vi "GEA2 Message to HEUI_LEDs_Idle.vi"(7 "Raw Data In":string) -> (8 "HEUI_LEDs":T1)   [LabVIEW 2016, in "TLMB.lvlib"]
uses:
  Projects/TLMB.lvlib
  controls/HEUI_LEDs.ctl
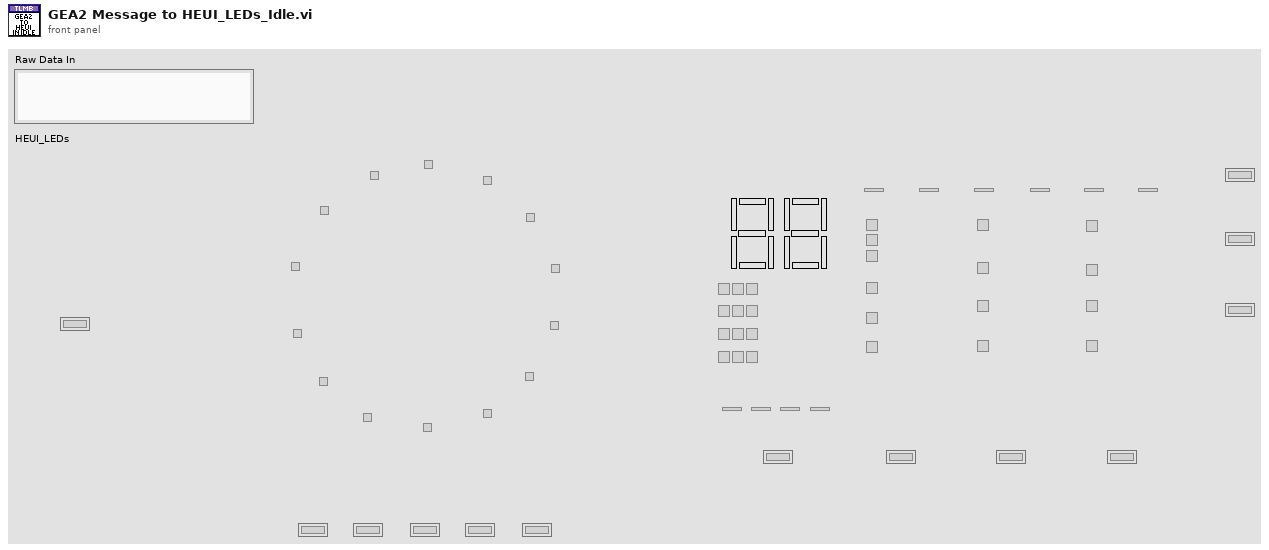
[diagram p1: front panel]
types:
  T1 = typedef "TLMB.lvlib/HEUI_LEDs.ctl" = cluster{"Z101 - Start":bool, "Z103 - Colors":bool, "Z104 - Whites":bool, "Z105 - Towels":bool, "Z106 - Bulky Items":bool, "Z107 - Heavy Duty":bool, "Z108 - Jeans":bool, "Z109 - Basket Clean":bool, "Z110 - Drain and Spin":bool, "Z111 - Rinse and Spin":bool, "Z112 - Speed Wash":bool, "Z113 - Active Wear":bool, "Z114 - Hand Wash":bool, "Z115 - Delicates":bool, "Z116 - Easy Care":bool, "Z117 - Tomato":bool, "Z118 - Wine":bool, "Z119 - Blood":bool, "Z120 - Grass":bool, "Z121 - Dirt":bool, "Z122_MSB_A":bool, "Z123_MSB_B":bool, "Z124_MSB_G":bool, "Z125_MSB_C":bool, "Z126_MSB_D":bool, "Z127_MSB_E":bool, "Z128_MSB_F":bool, "Z129_LSB_A":bool, "Z130_LSB_B":bool, "Z131_LSB_G":bool, "Z132_LSB_C":bool, "Z133_LSB_D":bool, "Z134_LSB_E":bool, "Z135_LSB_F":bool, "Z136 - Pause":bool, "Z137 - Pause":bool, "Z138 - Lock Controls":bool, "Z139 - Lock Controls":bool, "Z140 - Lock Controls":bool, "Z141 - Lid Lock":bool, "Z142 - Lid Lock":bool, "Z143 - Lid Lock":bool, "Z144 - Good":bool, "Z145":bool, "Z146":bool, "Z147 - Better":bool, "Z148 - Delay":bool, "Z149 - Fill":bool, "Z150 - Soak":bool, "Z151 - Wash":bool, "Z152 - Rinse":bool, "Z153 - Spin":bool, "Z154 - Hot":bool, "Z155 - Warm":bool, "Z156 - Colors":bool, "Z157 - Cool":bool, "Z158 - Cold":bool, "Z159 - Tap Cold":bool, "Z160 - Extra Heavy":bool, "Z161 - Heavy":bool, "Z162 - Normal":bool, "Z163 - Light":bool, "Z164 - Max Spin":bool, "Z165 - More Spin":bool, "Z166 - Normal Spin":bool, "Z167 - No Spin":bool, "Z168 - Extra Rinse":bool, "Z170 - Deep Rinse":bool, "Z171 - Auto Soak":bool, "Z172 - Warm Rinse":bool, "Z173 - Deep Fill":bool, "Z174 - My Cycles":bool, "Z175 - Delay Wash":bool, "Z176 - Spin Stop":bool, "Z177 - Spin Stop":bool, "Z178 - Spin Stop":bool, "Z179 - Pause":bool, "Z109":bool, "Z110":bool, "Z123":bool, "Z124":bool, "Z140":bool, "Unused0":bool, "Unused1":bool, "Unused2":bool, "Unused3":bool, "Channel_Off":bool, "Channel_Cycle_Unmapped":bool}
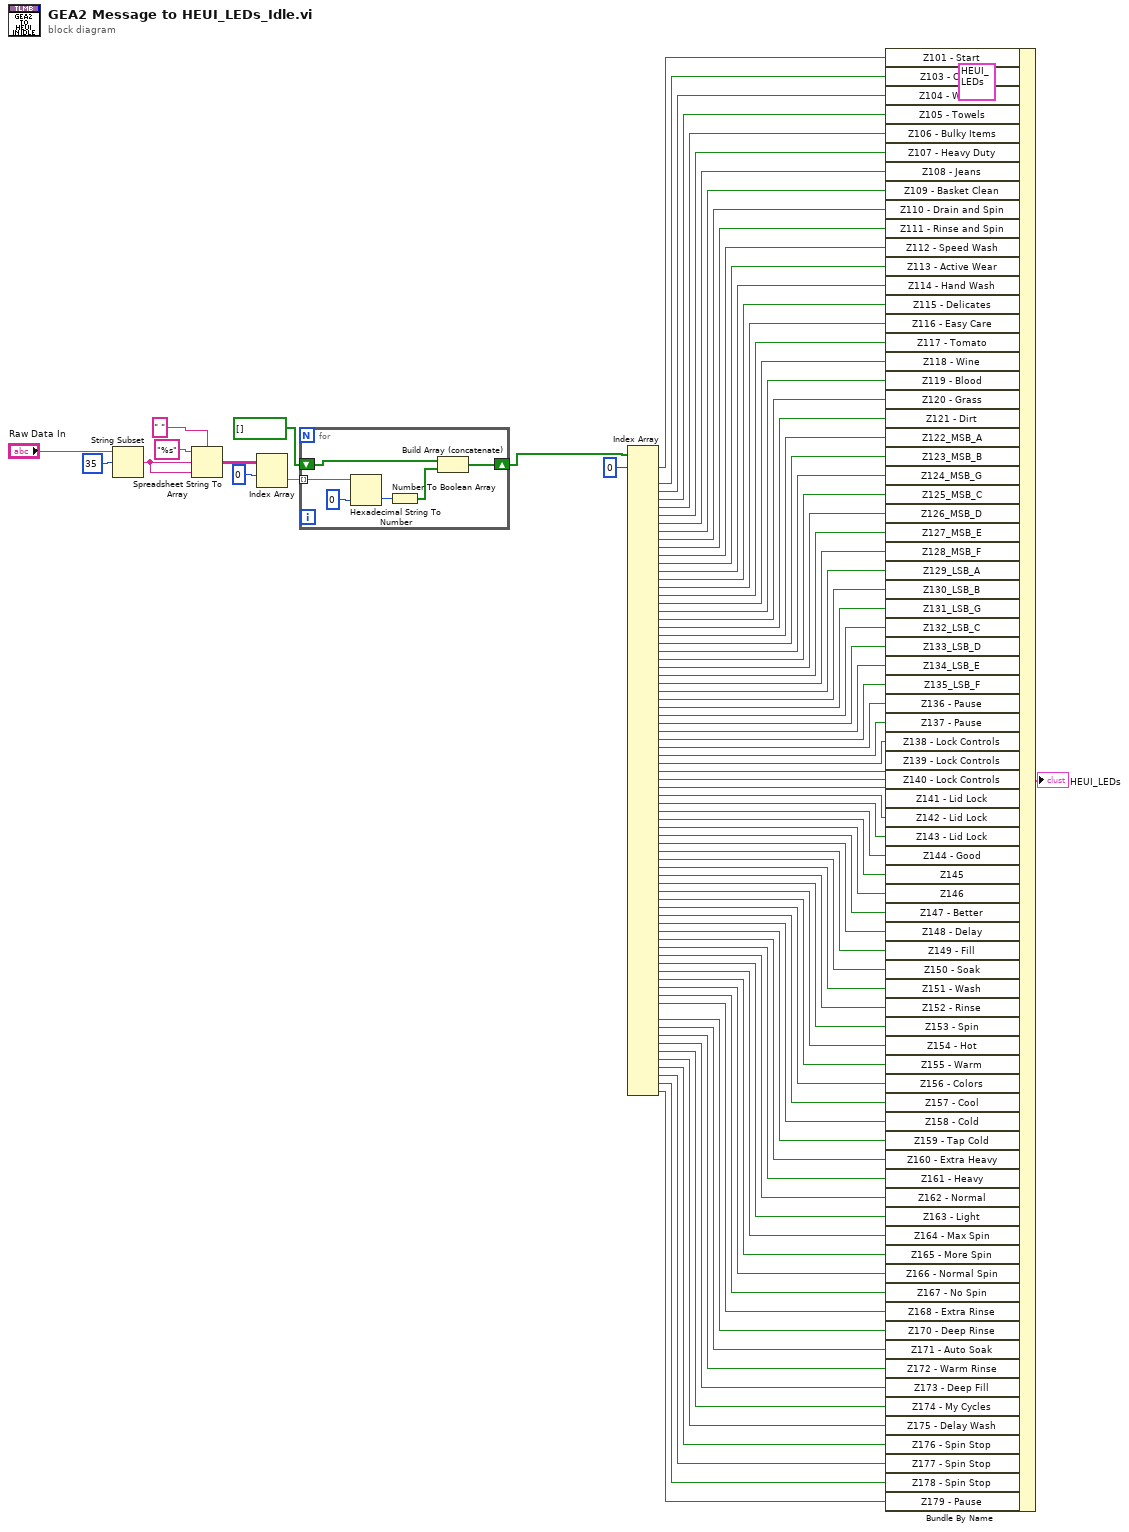
[diagram p0: block diagram]
diagram:
  n1 = String Subset(string="Raw Data In", offset (0)=35) -> (substring=w83:string)  [unwired: 1 in]
  n2 = Spreadsheet String To Array(delimiter (Tab)=" ", format string="%s", spreadsheet string=w83, array type (2D Dbl)=w83) -> (array=w87:string[][])
  n3 = Index Array(array=w87, index (row)=0) -> (element=w84:string[])  [unwired: 1 in]
  n4 = for {
    tunnel: w84 -> [w96] mode=indexing
    shift-right: [w92] -> w1
    shift-left: bool[] [] -> [w94]
    n5 = Hexadecimal String To Number(string=w96, default (0uL)=u8 0) -> (number=w95:u8)  [unwired: 1 in, 1 out]
    n6 = Number To Boolean Array(number=w95) -> (Boolean array=w93:bool[])
    n7 = Build Array (concatenate)(w94, w93) -> (w92:bool[])
  }
  n8 = Index Array(array=w1, index #1=0 ("index")) -> (element #1=w82:bool, element #3=w80:bool, element #4=w79:bool, element #5=w78:bool, element #6=w77:bool, element #7=w76:bool, element #8=w75:bool, element #9=w74:bool, element #10=w73:bool, element #11=w72:bool, element #12=w71:bool, element #13=w70:bool, element #14=w69:bool, element #15=w68:bool, element #16=w67:bool, element #17=w66:bool, element #18=w65:bool, element #19=w63:bool, element #20=w62:bool, element #21=w61:bool, element #22=w60:bool, element #23=w59:bool, element #24=w58:bool, element #25=w57:bool, element #26=w56:bool, element #27=w55:bool, element #28=w54:bool, element #29=w53:bool, element #30=w52:bool, element #31=w51:bool, element #32=w50:bool, element #33=w49:bool, element #34=w48:bool, element #35=w47:bool, element #36=w46:bool, element #37=w45:bool, element #38=w44:bool, element #39=w43:bool, element #40=w42:bool, element #41=w41:bool, element #42=w40:bool, element #43=w39:bool, element #44=w38:bool, element #45=w37:bool, element #46=w36:bool, element #47=w35:bool, element #48=w34:bool, element #49=w33:bool, element #50=w32:bool, element #51=w31:bool, element #52=w30:bool, element #53=w29:bool, element #54=w28:bool, element #55=w27:bool, element #56=w26:bool, element #57=w25:bool, element #58=w24:bool, element #59=w23:bool, element #60=w22:bool, element #61=w21:bool, element #62=w20:bool, element #63=w19:bool, element #64=w18:bool, element #65=w17:bool, element #66=w16:bool, element #67=w15:bool, element #68=w4:bool, element #70=w5:bool, element #71=w6:bool, element #72=w7:bool, element #73=w8:bool, element #74=w9:bool, element #75=w10:bool, element #76=w11:bool, element #77=w12:bool, element #78=w13:bool, element #79=w14:bool)  [unwired: 78 in, 2 out]
  n9 = Bundle By Name(cluster=T1 {"Z101 - Start"=FALSE, "Z103 - Colors"=FALSE, "Z104 - Whites"=FALSE, "Z105 - Towels"=FALSE, "Z106 - Bulky Items"=FALSE, "Z107 - Heavy Duty"=FALSE, "Z108 - Jeans"=FALSE, "Z109 - Basket Clean"=FALSE, "Z110 - Drain and Spin"=FALSE, "Z111 - Rinse and Spin"=FALSE, "Z112 - Speed Wash"=FALSE, "Z113 - Active Wear"=FALSE, "Z114 - Hand Wash"=FALSE, "Z115 - Delicates"=FALSE, "Z116 - Easy Care"=FALSE, "Z117 - Tomato"=FALSE, "Z118 - Wine"=FALSE, "Z119 - Blood"=FALSE, "Z120 - Grass"=FALSE, "Z121 - Dirt"=FALSE, "Z122_MSB_A"=FALSE, "Z123_MSB_B"=FALSE, "Z124_MSB_G"=FALSE, "Z125_MSB_C"=FALSE, "Z126_MSB_D"=FALSE, "Z127_MSB_E"=FALSE, "Z128_MSB_F"=FALSE, "Z129_LSB_A"=FALSE, "Z130_LSB_B"=FALSE, "Z131_LSB_G"=FALSE, "Z132_LSB_C"=FALSE, "Z133_LSB_D"=FALSE, "Z134_LSB_E"=FALSE, "Z135_LSB_F"=FALSE, "Z136 - Pause"=FALSE, "Z137 - Pause"=FALSE, "Z138 - Lock Controls"=FALSE, "Z139 - Lock Controls"=FALSE, "Z140 - Lock Controls"=FALSE, "Z141 - Lid Lock"=FALSE, "Z142 - Lid Lock"=FALSE, "Z143 - Lid Lock"=FALSE, "Z144 - Good"=FALSE, "Z145"=FALSE, "Z146"=FALSE, "Z147 - Better"=FALSE, "Z148 - Delay"=FALSE, "Z149 - Fill"=FALSE, "Z150 - Soak"=FALSE, "Z151 - Wash"=FALSE, "Z152 - Rinse"=FALSE, "Z153 - Spin"=FALSE, "Z154 - Hot"=FALSE, "Z155 - Warm"=FALSE, "Z156 - Colors"=FALSE, "Z157 - Cool"=FALSE, "Z158 - Cold"=FALSE, "Z159 - Tap Cold"=FALSE, "Z160 - Extra Heavy"=FALSE, "Z161 - Heavy"=FALSE, "Z162 - Normal"=FALSE, "Z163 - Light"=FALSE, "Z164 - Max Spin"=FALSE, "Z165 - More Spin"=FALSE, "Z166 - Normal Spin"=FALSE, "Z167 - No Spin"=FALSE, "Z168 - Extra Rinse"=FALSE, "Z170 - Deep Rinse"=FALSE, "Z171 - Auto Soak"=FALSE, "Z172 - Warm Rinse"=FALSE, "Z173 - Deep Fill"=FALSE, "Z174 - My Cycles"=FALSE, "Z175 - Delay Wash"=FALSE, "Z176 - Spin Stop"=FALSE, "Z177 - Spin Stop"=FALSE, "Z178 - Spin Stop"=FALSE, "Z179 - Pause"=FALSE, "Z109"=FALSE, "Z110"=FALSE, "Z123"=FALSE, "Z124"=FALSE, "Z140"=FALSE, "Unused0"=FALSE, "Unused1"=FALSE, "Unused2"=FALSE, "Unused3"=FALSE, "Channel_Off"=FALSE, "Channel_Cycle_Unmapped"=FALSE} ("HEUI_LEDs"), "Z101 - Start"=w82, "Z103 - Colors"=w80, "Z104 - Whites"=w79, "Z105 - Towels"=w78, "Z106 - Bulky Items"=w77, "Z107 - Heavy Duty"=w76, "Z108 - Jeans"=w75, "Z109 - Basket Clean"=w74, "Z110 - Drain and Spin"=w73, "Z111 - Rinse and Spin"=w72, "Z112 - Speed Wash"=w71, "Z113 - Active Wear"=w70, "Z114 - Hand Wash"=w69, "Z115 - Delicates"=w68, "Z116 - Easy Care"=w67, "Z117 - Tomato"=w66, "Z118 - Wine"=w65, "Z119 - Blood"=w63, "Z120 - Grass"=w62, "Z121 - Dirt"=w61, "Z122_MSB_A"=w60, "Z123_MSB_B"=w59, "Z124_MSB_G"=w58, "Z125_MSB_C"=w57, "Z126_MSB_D"=w56, "Z127_MSB_E"=w55, "Z128_MSB_F"=w54, "Z129_LSB_A"=w53, "Z130_LSB_B"=w52, "Z131_LSB_G"=w51, "Z132_LSB_C"=w50, "Z133_LSB_D"=w49, "Z134_LSB_E"=w48, "Z135_LSB_F"=w47, "Z136 - Pause"=w46, "Z137 - Pause"=w45, "Z138 - Lock Controls"=w44, "Z139 - Lock Controls"=w43, "Z140 - Lock Controls"=w42, "Z141 - Lid Lock"=w41, "Z142 - Lid Lock"=w40, "Z143 - Lid Lock"=w39, "Z144 - Good"=w38, "Z145"=w37, "Z146"=w36, "Z147 - Better"=w35, "Z148 - Delay"=w34, "Z149 - Fill"=w33, "Z150 - Soak"=w32, "Z151 - Wash"=w31, "Z152 - Rinse"=w30, "Z153 - Spin"=w29, "Z154 - Hot"=w28, "Z155 - Warm"=w27, "Z156 - Colors"=w26, "Z157 - Cool"=w25, "Z158 - Cold"=w24, "Z159 - Tap Cold"=w23, "Z160 - Extra Heavy"=w22, "Z161 - Heavy"=w21, "Z162 - Normal"=w20, "Z163 - Light"=w19, "Z164 - Max Spin"=w18, "Z165 - More Spin"=w17, "Z166 - Normal Spin"=w16, "Z167 - No Spin"=w15, "Z168 - Extra Rinse"=w4, "Z170 - Deep Rinse"=w5, "Z171 - Auto Soak"=w6, "Z172 - Warm Rinse"=w7, "Z173 - Deep Fill"=w8, "Z174 - My Cycles"=w9, "Z175 - Delay Wash"=w10, "Z176 - Spin Stop"=w11, "Z177 - Spin Stop"=w12, "Z178 - Spin Stop"=w13, "Z179 - Pause"=w14) -> (→"HEUI_LEDs":T1)
